vi "Device.compactDAQ.CheckConnect.vi"(7 "Devices in":T1, 8 "error in (no error)":errorcluster) -> (0 "error out":errorcluster, 3 "connect?":bool, 5 "Devices out":T1)   [LabVIEW 2019]
uses:
  Devices.ctl
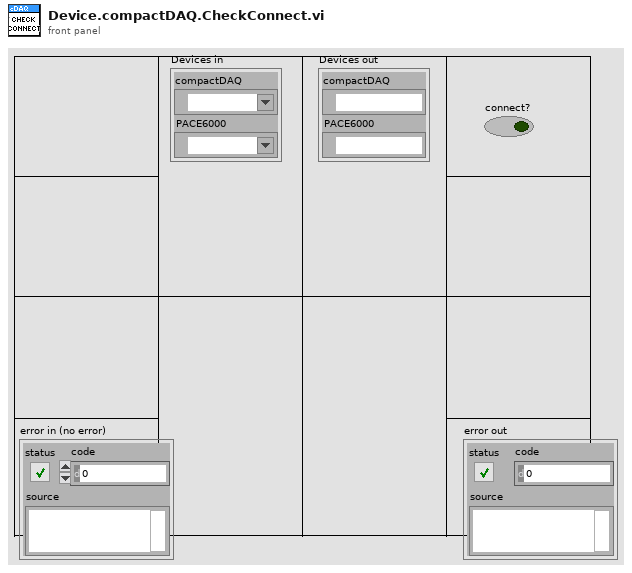
[diagram p1: front panel]
types:
  T1 = typedef "Devices.ctl" = cluster{"compactDAQ":tag, "PACE6000":refnum<visa-resource-name>}
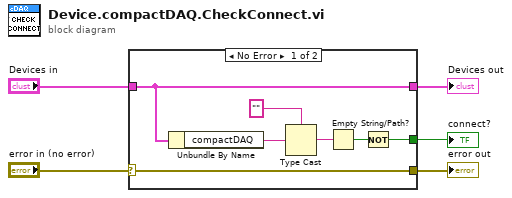
[diagram p0: block diagram]
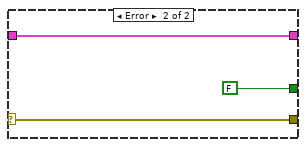
[diagram p2: hidden frame]
diagram:
  n1 = case shown="No Error" "error in (no error)" {
    selector: "error in (no error)" -> [w12 w15]
    tunnel: "Devices in" -> [w6 w13]
    tunnel: [w12 w15] -> w3
    tunnel: [w7 FALSE] -> w5
    tunnel: [w6 w13] -> w4
    frame No Error {
      n2 = Unbundle By Name(w6) -> ("compactDAQ"=w11:tag)
      n3 = Type Cast(type="", x=w11) -> (*(type *) &x=w9:string)
      n4 = Empty String/Path?(string/path=w9) -> (empty?=w8:bool)
      n5 = Not(x=w8) -> (.not. x?=w7:bool)
    }
    frame Error {
    }
  }
  "connect?" <- w5
  "Devices out" <- w4
  "error out" <- w3
